vi "Get Device Config_OLD.vi"(1 "Device ID":u8, 2 "Device Family":T4 items=["National Instruments", "Digilent", "Arduino"]) -> (0 "Device Config":T1)   [LabVIEW 2014, in "LMH-LINX.lvlib"]
uses:
  LMH-LINX.lvlib
  Type Defs/Device Family.ctl
  Type Defs/Devices/Generic Device.ctl
  Type Defs/Firmware Version.ctl
  Device/Type Defs/Firmware Interface.ctl
  Type Defs/Devices - NI.ctl
  Type Defs/Devices - Digilent.ctl
  Type Defs/Devices - Arduino.ctl
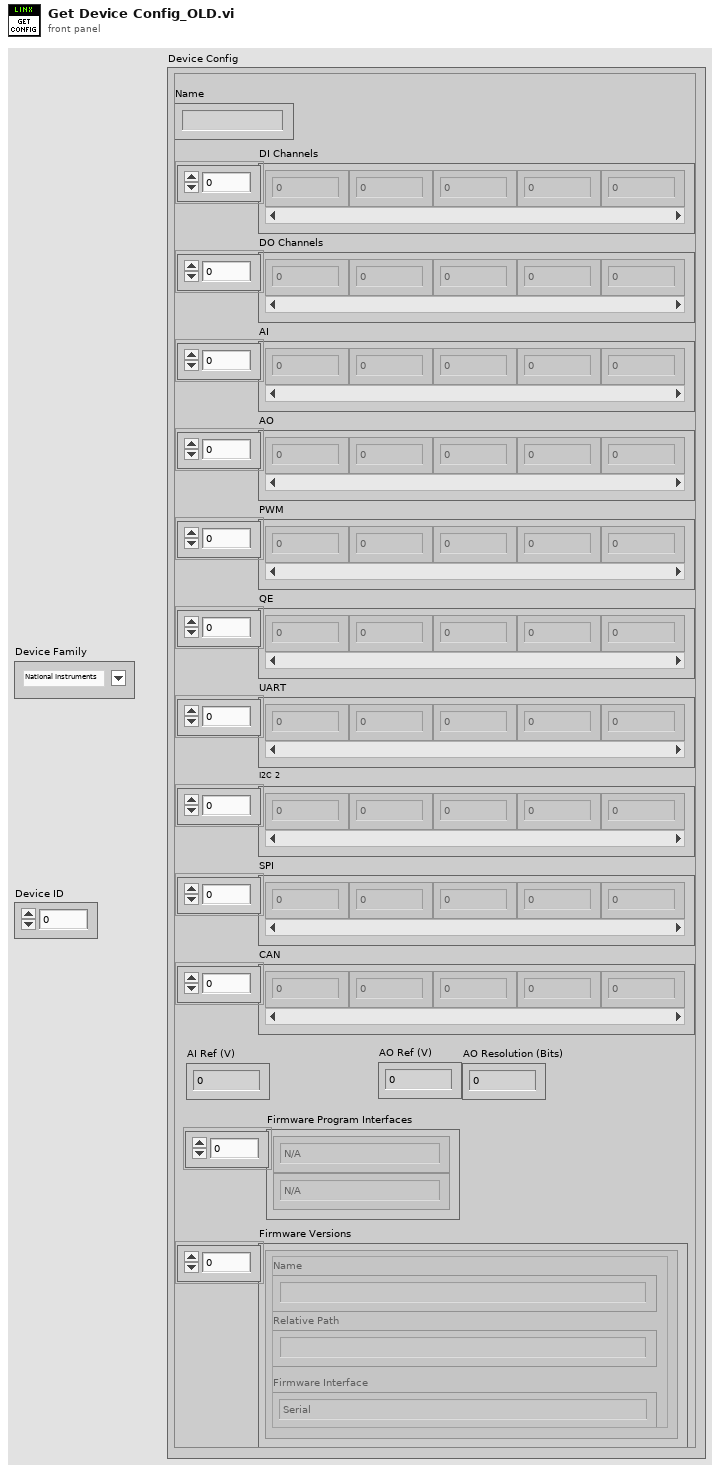
[diagram p1: front panel]
types:
  T1 = typedef "LMH-LINX.lvlib/Generic Device.ctl" = cluster{"DI Channels":u8[], "DO Channels":u8[], "AI":u8[], "AO":u8[], "PWM":u8[], "QE":u8[], "UART":u8[], "I2C 2":u8[], "SPI":u8[], "CAN":u8[], "AI Ref (V)":dbl, "Firmware Program Interfaces":enum16{"N/A", "Serial / USB", "USB", "TCP"}[], "Firmware Versions":T2[], "Name":string, "AO Resolution (Bits)":u8, "AO Ref (V)":dbl}
  T2 = typedef "LMH-LINX.lvlib/Firmware Version.ctl" = cluster{"Name":string, "Relative Path":string, "Firmware Interface":T3}
  T3 = typedef "LMH-LINX.lvlib/Firmware Interface.ctl" = enum32{"Serial ", "Ethernet", "WIFI"}
  T4 = typedef "LMH-LINX.lvlib/Device Family.ctl" = u8
  T5 = typedef "LMH-LINX.lvlib/Devices - NI.ctl" = enum16{"myRIO-1900", "myRIO-1950"}
  T6 = typedef "LMH-LINX.lvlib/Devices - Digilent.ctl" = enum16{"chipKIT Uno32", "chipKIT uC32", "chipKIT Max32", "chipKIT WF32"}
  T7 = typedef "LMH-LINX.lvlib/Devices - Arduino.ctl" = enum16{"Uno", "Mega 2560", "Leonardo", "Due", "Yun", "Nano", "Pro Mini", "Pro", "Fio", "Mega1280"}
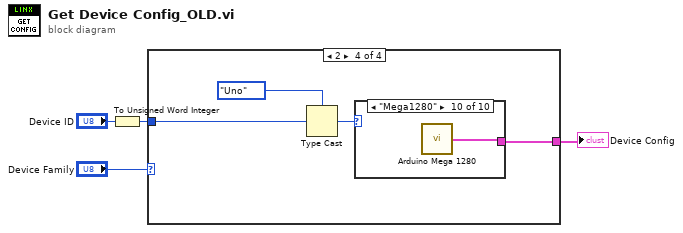
[diagram p0: block diagram]
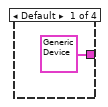
[diagram p2: hidden frame]
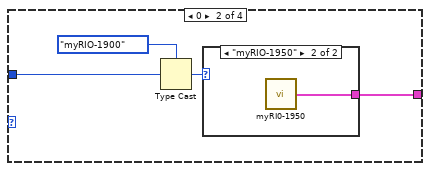
[diagram p3: hidden frame]
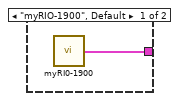
[diagram p4: hidden frame]
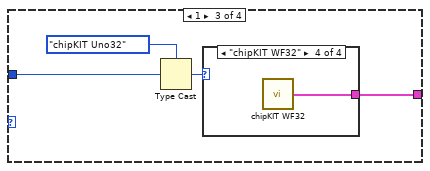
[diagram p5: hidden frame]
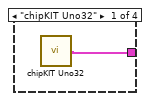
[diagram p6: hidden frame]
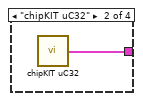
[diagram p7: hidden frame]
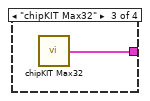
[diagram p8: hidden frame]
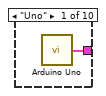
[diagram p9: hidden frame]
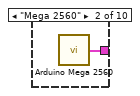
[diagram p10: hidden frame]
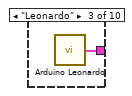
[diagram p11: hidden frame]
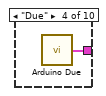
[diagram p12: hidden frame]
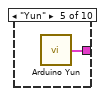
[diagram p13: hidden frame]
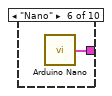
[diagram p14: hidden frame]
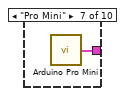
[diagram p15: hidden frame]
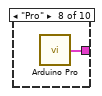
[diagram p16: hidden frame]
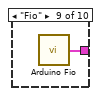
[diagram p17: hidden frame]
diagram:
  n1 = To Unsigned Word Integer(number="Device ID") -> (unsigned 16bit integer=w1:u16)
  n2 = case shown="2" "Device Family" {
    tunnel: [T1 {"DI Channels"=[], "DO Channels"=[], "AI"=[], "AO"=[], "PWM"=[], "QE"=[], "UART"=[], "I2C 2"=[], "SPI"=[], "CAN"=[], "AI Ref (V)"=0.0, "Firmware Program Interfaces"=[], "Firmware Versions"=[], "Name"="", "AO Resolution (Bits)"=0, "AO Ref (V)"=0.0} ("chipKIT DP32") w7 w14 w21] -> w3
    tunnel: w1 -> [_ w6 w12 w20]
    frame Default {
    }
    frame 0 {
      n3 = Type Cast(type=Devices_-_NI."myRIO-1900" ("NI Device"), x=w6) -> (*(type *) &x=w8:T5)
      n4 = case shown="\"myRIO-1950\"" w8 {
        tunnel: [w10 w11] -> w7
        frame "myRIO-1900", Default {
          n5 = call "myRI0-1900.vi"() -> ("myRIO-1900"=w10:T1)
        }
        frame "myRIO-1950" {
          n6 = call "myRI0-1950.vi"() -> ("myRIO-1950"=w11:T1)
        }
      }
    }
    frame 1 {
      n7 = Type Cast(type=Devices_-_Digilent."chipKIT Uno32" ("Digilent Device"), x=w12) -> (*(type *) &x=w15:T6)
      n8 = case shown="\"chipKIT WF32\"" w15 {
        tunnel: [w16 w17 w18 w19] -> w14
        frame "chipKIT Uno32" {
          n9 = call "chipKIT Uno32.vi"() -> ("chipKIT Uno32"=w16:T1)
        }
        frame "chipKIT uC32" {
          n10 = call "chipKIT uC32.vi"() -> ("chipKIT uC32"=w17:T1)
        }
        frame "chipKIT Max32" {
          n11 = call "chipKIT Max32.vi"() -> ("chipKIT Max32"=w18:T1)
        }
        frame "chipKIT WF32" {
          n12 = call "chipKIT WF32.vi"() -> ("chipKIT WF32"=w19:T1)
        }
      }
    }
    frame 2 {
      n13 = Type Cast(type=Devices_-_Arduino."Uno" ("Arduino Device"), x=w20) -> (*(type *) &x=w23:T7)
      n14 = case shown="\"Mega1280\"" w23 {
        tunnel: [w24 w25 w26 w27 w28 w29 w30 w31 w32 w33] -> w21
        frame "Uno" {
          n15 = call "Arduino Uno.vi"() -> ("Arduino Uno"=w24:T1)
        }
        frame "Mega 2560" {
          n16 = call "Arduino Mega 2560.vi"() -> ("Mega 2560"=w25:T1)
        }
        frame "Leonardo" {
          n17 = call "Arduino Leonardo.vi"() -> ("Arduino Leonardo"=w26:T1)
        }
        frame "Due" {
          n18 = call "Arduino Due.vi"() -> ("Due"=w27:T1)
        }
        frame "Yun" {
          n19 = call "Arduino Yun.vi"() -> ("Generic Device"=w28:T1)
        }
        frame "Nano" {
          n20 = call "Arduino Nano.vi"() -> ("Arduino Nano"=w29:T1)
        }
        frame "Pro Mini" {
          n21 = call "Arduino Pro Mini.vi"() -> ("Generic Device"=w30:T1)
        }
        frame "Pro" {
          n22 = call "Arduino Pro.vi"() -> ("Generic Device"=w31:T1)
        }
        frame "Fio" {
          n23 = call "Arduino Fio.vi"() -> ("Generic Device"=w32:T1)
        }
        frame "Mega1280" {
          n24 = call "Arduino Mega 1280.vi"() -> ("Mega 1280"=w33:T1)
        }
      }
    }
  }
  "Device Config" <- w3
